vi "Popup Complex Double.vi"(8 "error in (no error)":errorcluster, 9 "Panel":refnum<class "Panel.lvclass">, 10 "String in":string, 11 "Numeric Data Type in":refnum<class "Numeric Data Type.lvclass">) -> (0 "error out":errorcluster, 2 "String out":string, 3 "Numeric Data Type out":refnum<class "Numeric Data Type.lvclass">)   [LabVIEW 2018, in "Numeric Data Type.lvclass"]
uses:
  Numeric Data Type.lvclass
  <vilib>/MGI/Panel Manager/Panel/Panel/Panel.lvclass
  Numeric Data Type.lvclass/Numeric Data Type.ctl
  <vilib>/Utility/miscctls.llb/LVPointTypeDef.ctl
  String to Complex Number (CDB).vi
panel:
  in  "Numeric":cdb format="%.6e"
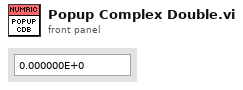
[diagram p1: front panel]
types:
  T1 = typedef "Numeric Data Type.lvclass/Response to Values Outside of Limits Enum.ctl" = enum16{"Ignore", "Coerce to nearest", "Coerce up", "Coerce down"}
  T2 = typedef "LVPointTypeDef.ctl" = cluster{"Horizontal":i16, "Vertical":i16}
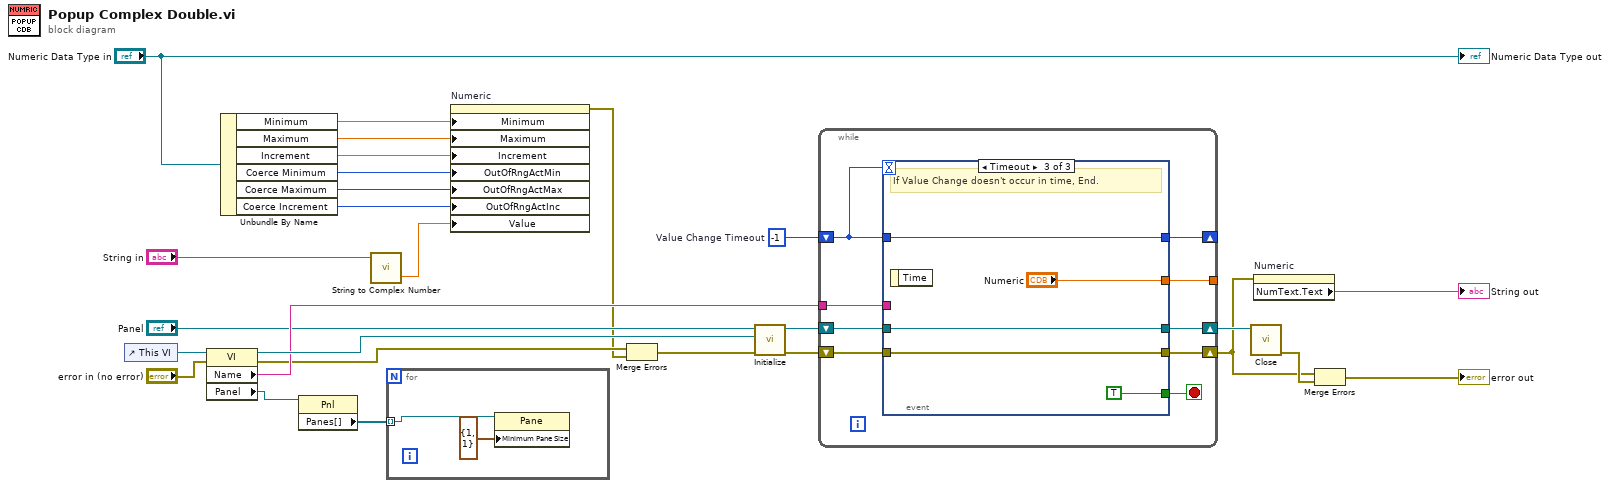
[diagram p0: block diagram]
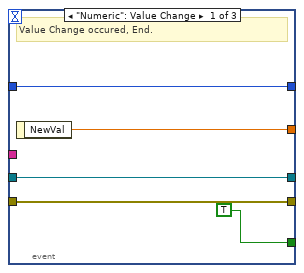
[diagram p2: hidden frame]
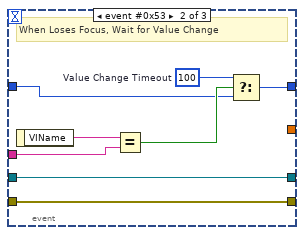
[diagram p3: hidden frame]
diagram:
  w27 = -1  # Value Change Timeout
  n1 = control-ref of="This VI"() -> (w24:refnum<vi>)
  n2 = property class="VI"(reference=w24, error in="error in (no error)") -> (reference out=w23:refnum<vi>, error out=w16:errorcluster, "Name"=w22:string, "Panel"=w6:refnum<vi>)
  n3 = Unbundle By Name("Numeric Data Type in") -> ("Minimum"=w15:dbl, "Maximum"=w14:dbl, "Increment"=w13:dbl, "Coerce Minimum"=w12:T1, "Coerce Maximum"=w11:T1, "Coerce Increment"=w10:T1)
  n4 = property class="Pnl"(reference=w6) -> ("Panes[]"=w5:refnum<vi>[])  [unwired: 1 in, 2 out]
  n5 = call-poly "String to Complex Number.vi"("string"="String in") -> ("number"=w3:cdb)  [unwired: 3 in, 1 out]
  n6 = for {
    tunnel: w5 -> [w29] mode=indexing
    n7 = property class="Pane"(reference=w29, "Minimum Pane Size"=T2 {"Horizontal"=1, "Vertical"=1}) -> ()  [unwired: 1 in, 2 out]
  }
  n8 = property on="Numeric" class="DigNum (strict)"("Minimum"=w15, "Maximum"=w14, "Increment"=w13, "OutOfRngActMin"=w12, "OutOfRngActMax"=w11, "OutOfRngActInc"=w10, "Value"=w3) -> (error out=w8:errorcluster)  [unwired: 2 in, 1 out]
  n9 = Merge Errors(w16, w8) -> (w9:errorcluster)
  n10 = call <vilib>:"Initialize.vi"("error in (no error)"=w9, "VI Refnum"=w23, "Panel In"="Panel") -> ("error out"=w25:errorcluster, "Panel Out"=w26:refnum<class "Panel.lvclass">)  [unwired: 6 in, 1 out]
  n11 = while {
    shift-right: [w38] -> w2
    shift-left: w25 -> [w37]
    shift-right: [w35] -> w20
    shift-left: w26 -> [w34]
    tunnel: [w33] -> _
    tunnel: w22 -> [w32]
    shift-right: [w30] -> _
    shift-left: w27 -> [w31]
    stop <- w36 stop-if-true
    n12 = event shown="[2] Timeout" {
      selector: _ -> [_ _ _]
      dyn-events: _ -> [_ _ _]
      timeout: w31 -> [_ _ _]
      tunnel: [w40 w49 w54] -> w38
      tunnel: w37 -> [w40 w49 w54]
      tunnel: [TRUE _ TRUE] -> w36
      tunnel: [w42 w48 w55] -> w35
      tunnel: w34 -> [w42 w48 w55]
      tunnel: [w41 _ "Numeric"] -> w33
      tunnel: w32 -> [_ w50 _]
      tunnel: w31 -> [w39 w45 w52]
      tunnel: [w39 w44 w52] -> w30
      event "Numeric": Value Change {
        # "Value Change occured, End."
        n13 = event-data() -> ("NewVal"=w41:cdb)  [unwired: 1 in]
      }
      event event #0x53 {
        w46 = 100  # Value Change Timeout
        # "When Loses Focus, Wait for Value Change"
        n14 = event-data() -> ("VIName"=w51:string)  [unwired: 1 in]
        n15 = Equal?(x=w51, y=w50) -> (x = y?=w47:bool)
        n16 = Select(t=w46, s=w47, f=w45) -> (s? t:f=w44:i32)
      }
      event Timeout {
        # "If Value Change doesn't occur in time, End."
        n17 = event-data() -> ()  [unwired: 1 in, 1 out]
      }
    }
  }
  n18 = call-dynamic "Close.vi"("Panel In"=w20) -> ("Error Out"=w21:errorcluster)  [unwired: 10 in]
  n19 = property on="Numeric" class="DigNum (strict)"(error in=w2) -> ("NumText.Text"=→"String out":string)  [unwired: 1 in, 2 out]
  n20 = Merge Errors(w2, w21) -> (→"error out":errorcluster)
  "Numeric Data Type out" <- "Numeric Data Type in"
